vi "write_upconfig.vi"(0 "object in":refnum<class "interface.lvclass">, 1 "段":string="应用程序交互", 2 "键数组":string[](array[string]), 3 "configuration file path":path caption="配置文件的路径", 4 "updateconfiguration":T1={"主机"="27.154.58.30", "用户"="update", "密码"="std23506", "远程路径"="数据传输系统\\平台数据传输系统.exe", "下载文件名"="数据传输系统.exe", "软件版本"=""}, 5 "error in (no error)":errorcluster) -> (14 "object out":refnum<class "interface.lvclass">, 19 "error out":errorcluster)   [LabVIEW 2016, in "interface.lvclass"]
uses:
  interface.lvclass
  <vilib>/Utility/config.llb/Write Key (I32).vi
  <vilib>/Utility/config.llb/Write Key (String).vi
  <vilib>/Utility/Data Type/NI_Data Type.lvlib
  <vilib>/Utility/config.llb/NI_LVConfig.lvlib
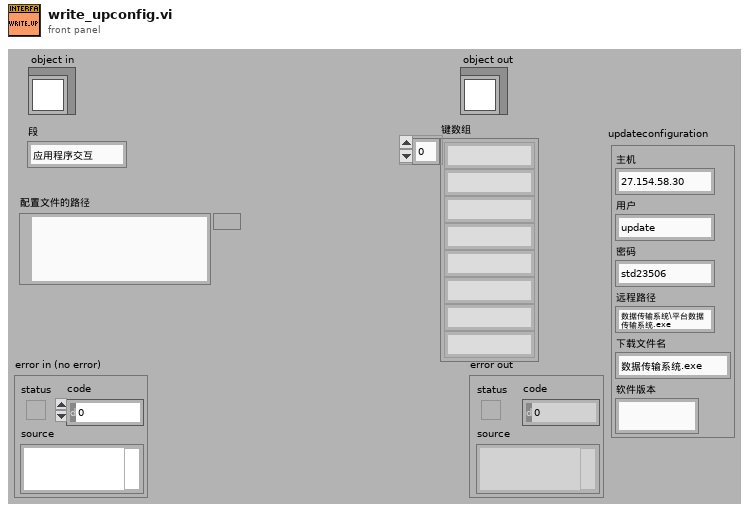
[diagram p1: front panel]
types:
  T1 = cluster{"主机":string, "用户":string, "密码":string, "远程路径":string, "下载文件名":string, "软件版本":string}
  T2 = typedef "NI_LVConfig.lvlib/Config Data RefNum.ctl" = refnum<k1>
  T3 = typedef "NI_Data Type.lvlib/Data Type.ctl" = enum8{"Invalid Type", "Void", "I8", "I16", "I32", "I64", "U8", "U16", "U32", "U64", "Single Float", "Double Float", "Extended Float", "Single Complex", "Double Complex", "Extended Complex", "Enum U8", "Enum U16", "Enum U32", "Enum U64", "Single Float With Unit", "Double Float With Unit", "Extended Float With Unit", "Single Complex with Unit", "Double Complex with Unit", "Extended Complex with Unit", "Boolean", "String", "Path", "Picture", "Tag", "Array", "Cluster", "Variant", "LV Variant", "Waveform", "Timestamp", "Digital Waveform", "Digital Data", "ExpressData", "Refnum", "External Data", "VI", "Poly VI", "LabVIEW Class Instance", "Fixed Point"}
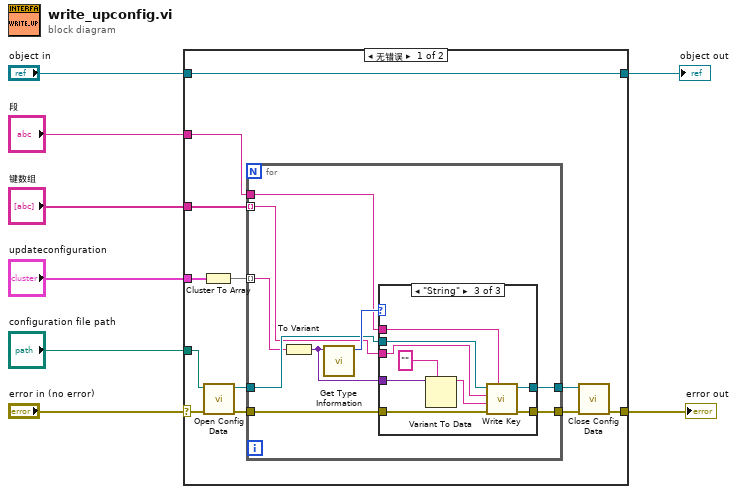
[diagram p0: block diagram]
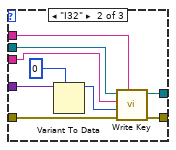
[diagram p3: hidden frame]
diagram:
  n1 = case shown="无错误" "error in (no error)" {
    selector: "error in (no error)" -> [w9 w51]
    tunnel: [w10 w51] -> w7
    tunnel: [w20 w50] -> w5
    tunnel: "object in" -> [w20 w50]
    tunnel: "段" -> [w14 _]
    tunnel: "键数组" -> [w13 _]
    tunnel: "updateconfiguration" -> [w12 _]
    tunnel: "configuration file path" -> [w11 _]
    frame No Error {
      n2 = Cluster To Array(cluster=w12) -> (array=w19:string[])
      n3 = call <vilib>:"Open Config Data.vi"("error in (no error)"=w9, "configuration file path"=w11) -> ("error out"=w16:errorcluster, "refnum"=w15:T2)  [unwired: 7 in, 1 out]
      n4 = for {
        tunnel: w13 -> [w25] mode=indexing
        tunnel: w19 -> [w22] mode=indexing
        tunnel: w15 -> [w28]
        tunnel: w16 -> [w27]
        tunnel: w14 -> [w26]
        tunnel: [w24] -> w17
        tunnel: [w23] -> w18
        n5 = To Variant(anything=w22) -> (Variant=w21:variant)
        n6 = call <vilib>:"Get Type Information.vi"("Variant"=w21) -> ("Type"=w29:T3)  [unwired: 6 in, 4 out]
        n7 = case shown="\"String\"" w29 {
          tunnel: [w31 w38 w47] -> w24
          tunnel: [w30 w37 w46] -> w23
          tunnel: w21 -> [_ w32 w45]
          tunnel: w28 -> [w31 w36 w44]
          tunnel: w27 -> [w30 w35 w43]
          tunnel: w26 -> [_ w34 w42]
          tunnel: w25 -> [_ w33 w41]
          frame "Invalid Type", Default {
          }
          frame "I32" {
            n8 = Variant To Data(type=0, Variant=w32) -> (data=w39:i32)  [unwired: 1 in, 1 out]
            n9 = call-poly <vilib>:"Write Key.vi"("section"=w34, "error in (no error)"=w35, "value"=w39, "key"=w33, "refnum"=w36) -> ("error out"=w37:errorcluster, "refnum out"=w38:T2)  [unwired: 4 in, 1 out]
          }
          frame "String" {
            n10 = Variant To Data(type="", Variant=w45) -> (data=w48:string)  [unwired: 1 in, 1 out]
            n11 = call-poly <vilib>:"Write Key.vi"("section"=w42, "error in (no error)"=w43, "value"=w48, "key"=w41, "refnum"=w44) -> ("error out"=w46:errorcluster, "refnum out"=w47:T2)  [unwired: 4 in, 1 out]
          }
        }
      }
      n12 = call <vilib>:"Close Config Data.vi"("error in (no error)"=w18, "refnum"=w17) -> ("error out"=w10:errorcluster)  [unwired: 8 in, 1 out]
    }
    frame Error {
    }
  }
  "error out" <- w7
  "object out" <- w5
